vi "result ng check.vi"(11 "MSG":T1) -> (1 "PART OK REMOVE PART":bool, 3 "Result NG":bool)   [LabVIEW 2015]
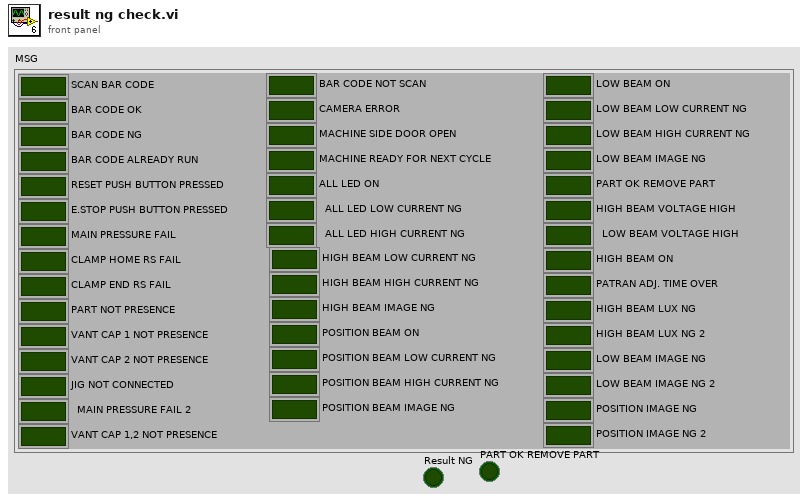
[diagram p1: front panel]
types:
  T1 = cluster{"SCAN BAR CODE":bool, "BAR CODE OK":bool, "BAR CODE NG":bool, "BAR CODE ALREADY RUN":bool, "RESET PUSH BUTTON PRESSED":bool, "E.STOP PUSH BUTTON PRESSED":bool, "MAIN PRESSURE FAIL":bool, "CLAMP HOME RS FAIL":bool, "CLAMP END RS FAIL ":bool, "PART NOT PRESENCE ":bool, "VANT CAP 1 NOT PRESENCE":bool, "VANT CAP 2 NOT PRESENCE":bool, "JIG NOT CONNECTED":bool, "\tMAIN PRESSURE FAIL 2":bool, "VANT CAP 1,2 NOT PRESENCE":bool, "BAR CODE NOT SCAN":bool, "CAMERA ERROR ":bool, "MACHINE SIDE DOOR OPEN":bool, "MACHINE READY FOR NEXT CYCLE":bool, "ALL LED ON ":bool, "\tALL LED LOW CURRENT NG":bool, "\tALL LED HIGH CURRENT NG":bool, "HIGH BEAM LOW CURRENT NG":bool, "HIGH BEAM HIGH CURRENT NG":bool, "HIGH BEAM IMAGE NG":bool, "POSITION BEAM ON ":bool, "POSITION BEAM LOW CURRENT NG":bool, "POSITION BEAM HIGH CURRENT NG":bool, "POSITION BEAM IMAGE NG":bool, "LOW BEAM ON":bool, "LOW BEAM LOW CURRENT NG":bool, "LOW BEAM HIGH CURRENT NG":bool, "LOW BEAM IMAGE NG":bool, "PART OK REMOVE PART ":bool, "HIGH BEAM VOLTAGE HIGH":bool, "\tLOW BEAM VOLTAGE HIGH":bool, "HIGH BEAM ON":bool, "PATRAN ADJ. TIME OVER":bool, "HIGH BEAM LUX NG ":bool, "HIGH BEAM LUX NG 2":bool, "LOW BEAM IMAGE NG":bool, "LOW BEAM IMAGE NG 2":bool, "POSITION IMAGE NG":bool, "POSITION IMAGE NG 2":bool}
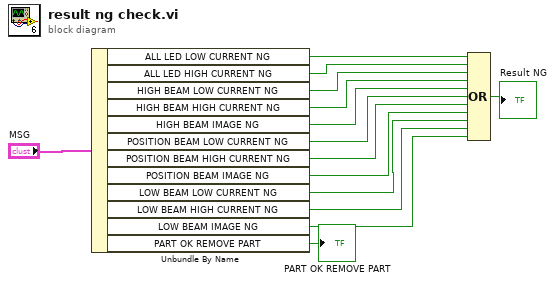
[diagram p0: block diagram]
diagram:
  n1 = Unbundle By Name("MSG") -> ("ALL LED LOW CURRENT NG"=w13:bool, "ALL LED HIGH CURRENT NG"=w12:bool, "HIGH BEAM LOW CURRENT NG"=w11:bool, "HIGH BEAM HIGH CURRENT NG"=w10:bool, "HIGH BEAM IMAGE NG"=w9:bool, "POSITION BEAM LOW CURRENT NG"=w8:bool, "POSITION BEAM HIGH CURRENT NG"=w7:bool, "POSITION BEAM IMAGE NG"=w6:bool, "LOW BEAM LOW CURRENT NG"=w5:bool, "LOW BEAM HIGH CURRENT NG"=w4:bool, "LOW BEAM IMAGE NG"=w3:bool, "PART OK REMOVE PART"=→"PART OK REMOVE PART":bool)
  n2 = Compound Arithmetic op=OR(w13, w12, w11, w10, w9, w8, w7, w6, w5, w4, w3) -> (→"Result NG":bool)
